vi "Control Panel Global.vi"() -> ()   [LabVIEW 2019]
panel:
  out "Boolean":bool
  in  "Counter":dbl
  in  "Motor Speed":dbl=0.5
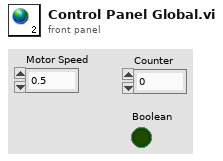
[diagram p1: front panel]
diagram:
